vi "Stop Core.vi"(10 "final error code":i32, 11 "Master Controller in":refnum<class "EMS User Interface.lvclass">) -> (3 "Master Controller out":refnum<class "EMS User Interface.lvclass">)   [LabVIEW 2018, in "EMS User Interface Actor.lvlib" / "EMS User Interface.lvclass"]
doc: "(<B>Filename</B>: Actor Framework.lvlib:Actor.lvclass:Stop Core.vi)\n\nDefines what the actor does before it stops. Use the <B>final error code</B> input to determine whether the actor shut down in response to an error.\n\nBy default, this method does nothing. A descendant class may override it to define behavior, such as shutting down any processes the actor initiated in its override of the Actor Core method."
uses:
  EMS User Interface.lvclass
  C:/Users/Administrator/Desktop/2018LabVIEW EMS/EMS Generic Actor/EMS Generic/EMS Generic.lvclass
  EMS User Interface.lvclass/EMS User Interface.ctl
  <vilib>/ActorFramework/Message Enqueuer/Message Enqueuer.lvclass/Message Enqueuer.ctl
  <vilib>/ActorFramework/Message Enqueuer/Enqueue.vi
  <vilib>/ActorFramework/Stop Msg/Stop Msg.lvclass
  C:/Program Files (x86)/National Instruments/LabVIEW 2018/vi.lib/ActorFramework/Message/Message.lvclass
  <vilib>/ActorFramework/Message Priority Queue/Priority Enqueue.vi
  EMS Generic Actor/EMS Generic/EMS Generic.lvclass
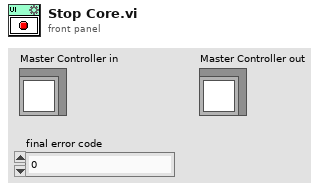
[diagram p1: front panel]
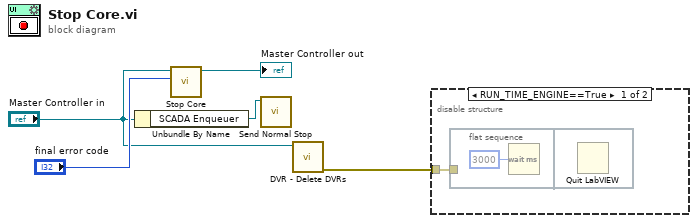
[diagram p0: block diagram]
diagram:
  n1 = Unbundle By Name("Master Controller in") -> ("SCADA Enqueuer"=w3:refnum<class "Message Enqueuer.lvclass">)
  n2 = call-parent "Stop Core.vi"("final error code"="final error code", "EMS Generic in"="Master Controller in") -> ("EMS Generic out"=→"Master Controller out":refnum<class "EMS User Interface.lvclass">)  [unwired: 9 in]
  n3 = call <vilib>:"Send Normal Stop.vi"("Message Enqueuer"=w3) -> ()  [unwired: 10 in, 1 out]
  n4 = call "DVR - Delete DVRs.vi"("EMS Generic in"="Master Controller in") -> ("error out"=w1:errorcluster)  [unwired: 9 in, 1 out]
  n5 = disable-structure shown="RUN_TIME_ENGINE==True" {
    disable-tunnel: w1 -> [w6 _]
    frame condition #0 {
      n6 = flat-sequence {
        tunnel: w6 -> [_]
        frame #0 {
          n7 = Wait (ms)(milliseconds to wait=u32 3000) -> ()  [unwired: 1 out]
        }
        frame #1 {
          n8 = Quit LabVIEW() -> ()  [unwired: 1 in]
        }
      }
    }
    frame condition #1 (active) {
    }
  }
